vi "rule editor.vi"() -> (0 "output descriptions out":string[][](array[string]), 1 "State names":string[](array[string]), 3 "rule file":path, 4 "output descriptions out 2":string[][](array[string]))   [LabVIEW 2015]
uses:
  rule.ctl
  condition.ctl
  greater or less.ctl
  toolbar icons/Save configuration.ctl
  toolbar icons/open configuration.ctl
  toolbar icons/help.ctl
  variable setpoint.ctl
  data ave interval.ctl
  type specifier for control code.ctl
  rules.ctl
  State rules.ctl
  Output control.ctl
  logic buffer cmd.ctl
  Calibration and Function folders.ctl
  DAQ configuration/Sensor buffer command.ctl
  calibration/Shared Data/share data command.ctl
  <vilib>/Platform/browser.llb/Open URL in Default Browser (string).vi
panel:
  in  "new element/subarray":T1={"name"="new set point", "unit"="", "value"=0.0, "Type"=enum."Constant", "variable"={"selected sensors"=[], "selected set points"=[], "VI"=path "", "Data average interval"=0.0, "code ref"=refnum}} {"value" format="%#_6p"; "variable"."Data average interval" min=0.0 format="%^#_3g"}
  in  "Tab Control":enum32{"Set Points", "Rules & Outputs"}(tab)
  in  "Delete all set points":bool
  in  "Configure Function":bool
  in  "Calculate set point":bool
  out "Required Sensors":i32(listbox)
  out "Required Set Points":i32(listbox)
  out "code match":bool
  out "data match":bool
  in  "S P & V definitions":T1[](array[typedef]) {"value" format="%#_6p"; "variable"."Data average interval" min=0.0 format="%^#_3g"}
  in  "delete set point":bool
  in  "add set point after":bool
  in  "Set Points and Variables List":i32(listbox)=1
  in  "Tab states and rules":enum32{"Rules", "Outputs"}(tab)
  in  "Rules":T4=[{"state rules"=[{"next state"=0, "conditions"=[], "number of conditions"=0, "Rule name"=""}, {"next state"=1, "conditions"=[{"> or <"=FALSE, "set point"=500, "sensors and variables"=0, "Data average interval"=0.0}], "number of conditions"=1, "Rule name"=""}, {"next state"=1, "conditions"=[{"> or <"=FALSE, "set point"=10, "sensors and variables"=0, "Data average interval"=0.0}, {"> or <"=FALSE, "set point"=10, "sensors and variables"=0, "Data average interval"=0.0}, {"> or <"=TRUE, "set point"=20, "sensors and variables"=0, "Data average interval"=0.0}, {"> or <"=TRUE, "set point"=500, "sensors and variables"=0, "Data average interval"=0.0}], "number of conditions"=4, "Rule name"=""}], "State name"=""}, {"state rules"=[{"next state"=1, "conditions"=[{"> or <"=FALSE, "set point"=0, "sensors and variables"=0, "Data average interval"=0.0}], "number of conditions"=1, "Rule name"=""}, {"next state"=0, "conditions"=[{"> or <"=FALSE, "set point"=0, "sensors and variables"=0, "Data average interval"=0.0}], "number of conditions"=4, "Rule name"=""}], "State name"=""}] {"state rules"."number of conditions" min=1 step=1; "state rules"."conditions"."Data average interval" min=0.0 format="%^#_3g"; "state rules"."conditions"."sensors and variables" items=["Elapsed time in current state"]; "state rules"."conditions"."set point" items=["OFF", "ON"]; "state rules"."next state" items=["OFF"]}
  in  "output descriptions":string[][](array[string])
  in  "output settings":T9 items=["OFF", "ON"]
  in  "delete rule":bool
  in  "add rule after":bool
  in  "Rule List":i32(listbox)
  in  "delete state":bool
  in  "add state after":bool
  in  "State List":i32(listbox)
  in  "Help Button":T10
  out "Sensor names":string[](array[string])
  in  "Open logic":T11
  in  "Save logic":T12
  in  "new rule":cluster{"state rules":T6[], "State name":string}={"state rules"=[{"next state"=0, "conditions"=[{"> or <"=FALSE, "set point"=0, "sensors and variables"=0, "Data average interval"=0.0}], "number of conditions"=1, "Rule name"="New Rule"}], "State name"="New State"} {"state rules"."number of conditions" min=1 step=1; "state rules"."conditions"."Data average interval" min=0.0 format="%^#_3g"; "state rules"."conditions"."sensors and variables" items=["Elapsed time in current state"]; "state rules"."next state" items=["john", "dick"]}
  in  "OK Button":bool
  out "Unit":string[](array[string])
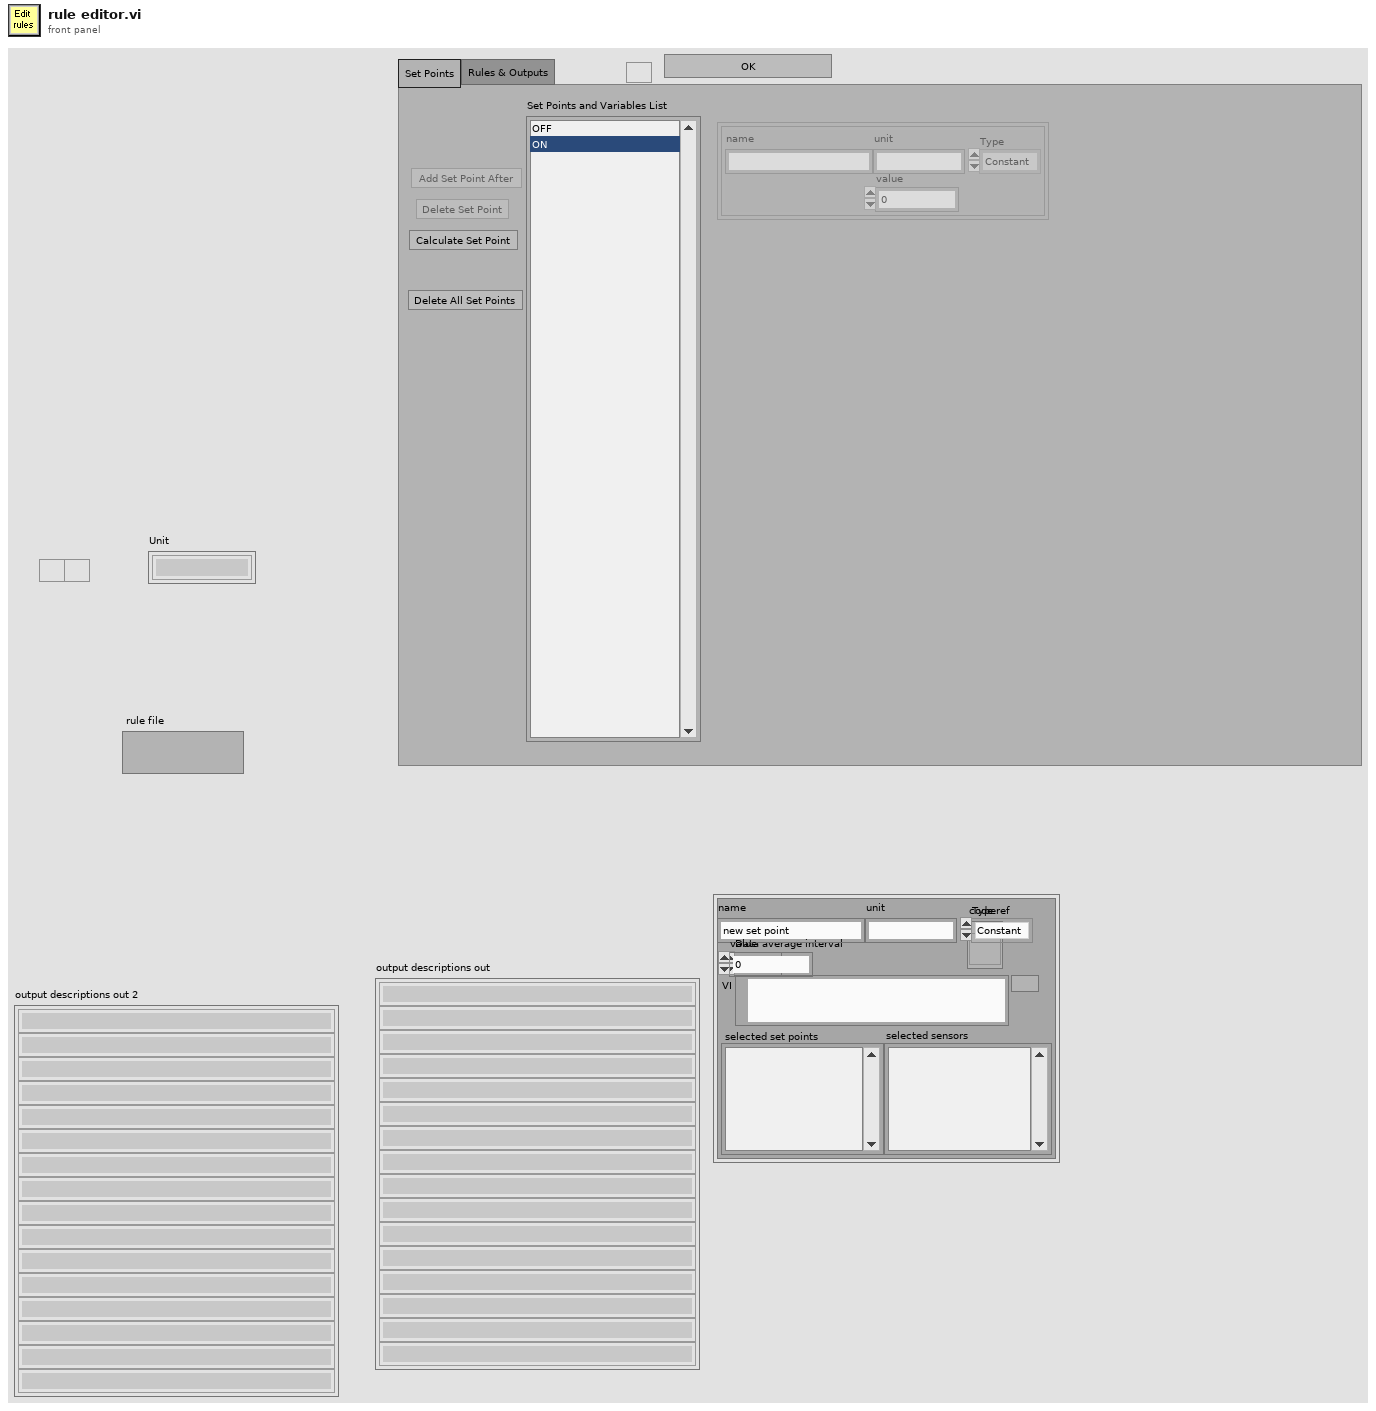
[diagram p1: front panel]
types:
  T1 = typedef "variable setpoint.ctl" = cluster{"name":string, "unit":string, "value":dbl, "Type":enum16{"Constant", "Variable"}, "variable":cluster{"selected sensors":i32[], "selected set points":i32[], "VI":path, "Data average interval":T2, "code ref":T3}}
  T2 = typedef "data ave interval.ctl" = dbl
  T3 = typedef "type specifier for control code.ctl" = refnum<vi>
  T4 = typedef "rules.ctl" = T5[]
  T5 = typedef "State rules.ctl" = cluster{"state rules":T6[], "State name":string}
  T6 = typedef "rule.ctl" = cluster{"next state":u16, "conditions":T7[], "number of conditions":u8, "Rule name":string}
  T7 = typedef "condition.ctl" = cluster{"> or <":T8, "set point":i32, "sensors and variables":i32, "Data average interval":dbl}
  T8 = typedef "greater or less.ctl" = bool
  T9 = typedef "Output control.ctl" = u16[][]
  T10 = typedef "help.ctl" = bool
  T11 = typedef "open configuration.ctl" = bool
  T12 = typedef "Save configuration.ctl" = bool
  T13 = typedef "share data command.ctl" = enum16{"Initialize from ini", "Update ini", "Write data", "Read data", "List my data", "List shared data", "Close"}
  T14 = typedef "Sensor buffer command.ctl" = enum16{"read average", "read recent", "read all", "write", "set buffer size", "Read channel config", "Write channel config", "clear"}
  T15 = typedef "Calibration and Function folders.ctl" = enum16{"Sensors", "Functions", "Config File", "PublicAppFolder", "New ini File", "Set Config File", "Delete ini File"}
  T16 = typedef "logic buffer cmd.ctl" = enum16{"read", "write ouput settings", "write rules", "write setpoints", "write output descriptions", "write all", "calculate setpoints", "save", "open", "Load all setpoint code", "Load one setpoint code", "Configure one setpoint code"}
  T17 = typedef "setpoint match.ctl" = cluster{"required data":cluster{"Set Point names":string[], "required number of setpoints":u8, "required number of sensors":u8, "Sensor names":string[]}, "input match":bool, "code match":bool, "variable?":bool}
  T18 = typedef "Channel config.ctl" = cluster{"Channel Indices":T19[], "AI Max voltage":dbl[], "Calibration matrix":T20}
  T19 = typedef "channel identifier.ctl" = u16
  T20 = typedef "calib array.ctl" = T21[]
  T21 = typedef "conversion.ctl" = cluster{"conversion matrix":sgl[][], "units":string, "name":string, "scale type":T22, "offset (volts)":dbl, "second channel":i8, "correspondence table":T23, "offset (physical units)":dbl, "pH scale":T24, "D.O.":T25, "Photometer data":T26}
  T22 = typedef "scale type.ctl" = enum16{"Volts", "Polynomial", "Correspondence Table", "pH", "Dissolved Oxygen", "Quadratic", "Photometer"}
  T23 = typedef "correspondence table.ctl" = cluster{"physical units":dbl, "volts":dbl}[]
  T24 = typedef "pH scale.ctl" = cluster{"Buffers":cluster{"Buffer":dbl, "Calibrated":bool, "V/T":dbl}[], "Temperature":dbl}
  T25 = typedef "DO scale.ctl" = cluster{"Temperature":dbl, "K":dbl, "barometric pressure":dbl}
  T26 = typedef "Photometer calibration data.ctl" = cluster{"Dark Voltage":dbl, "Blank Voltage":dbl, "Standards":cluster{"Concentration":dbl, "Voltage":dbl}[]}
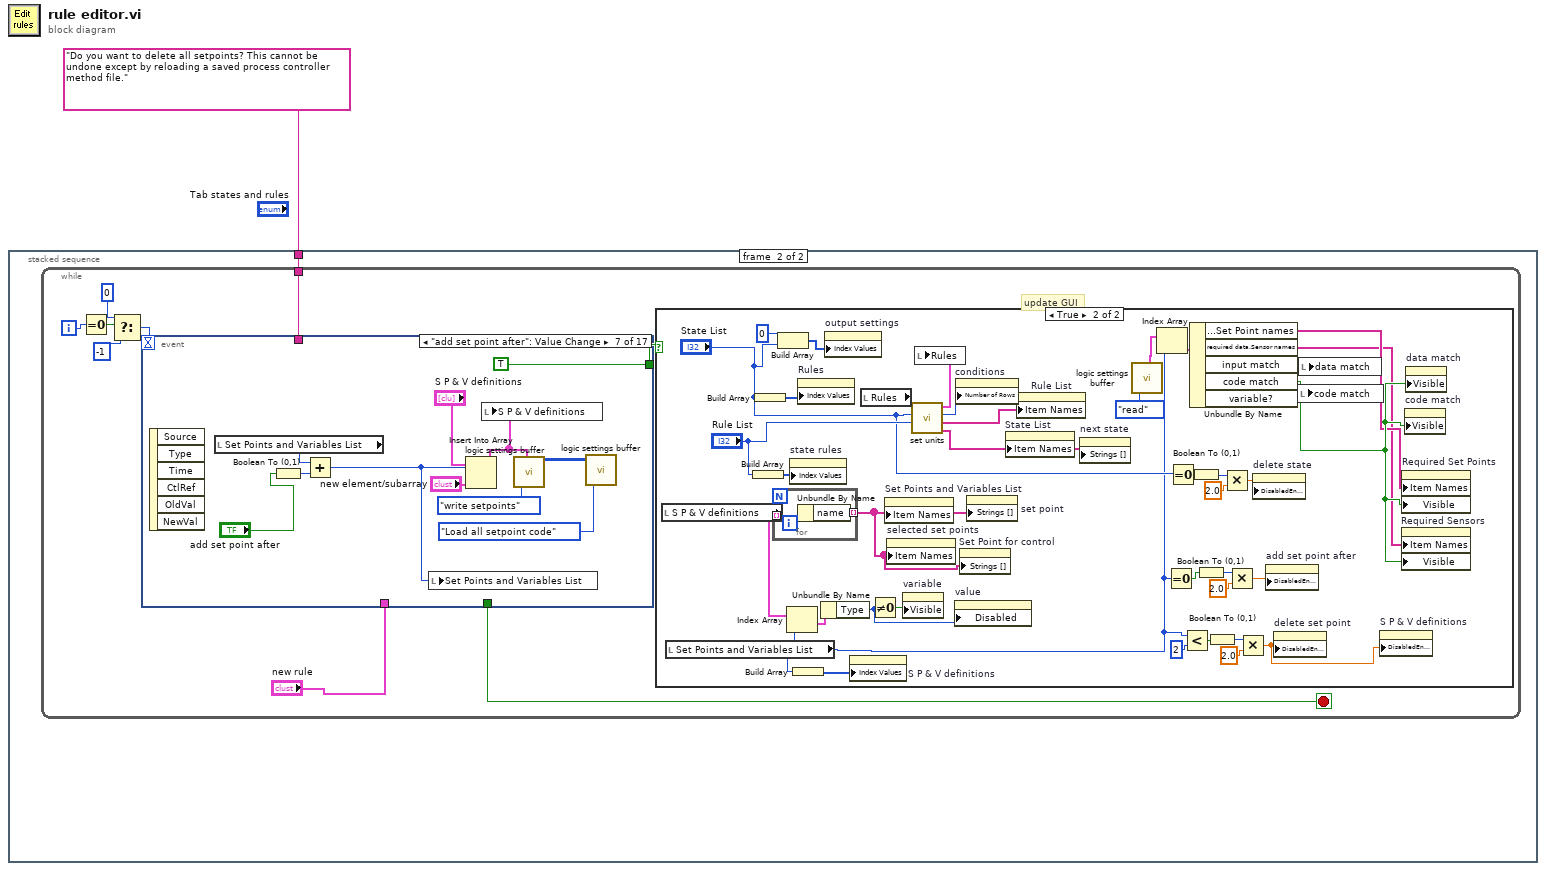
[diagram p0: block diagram]
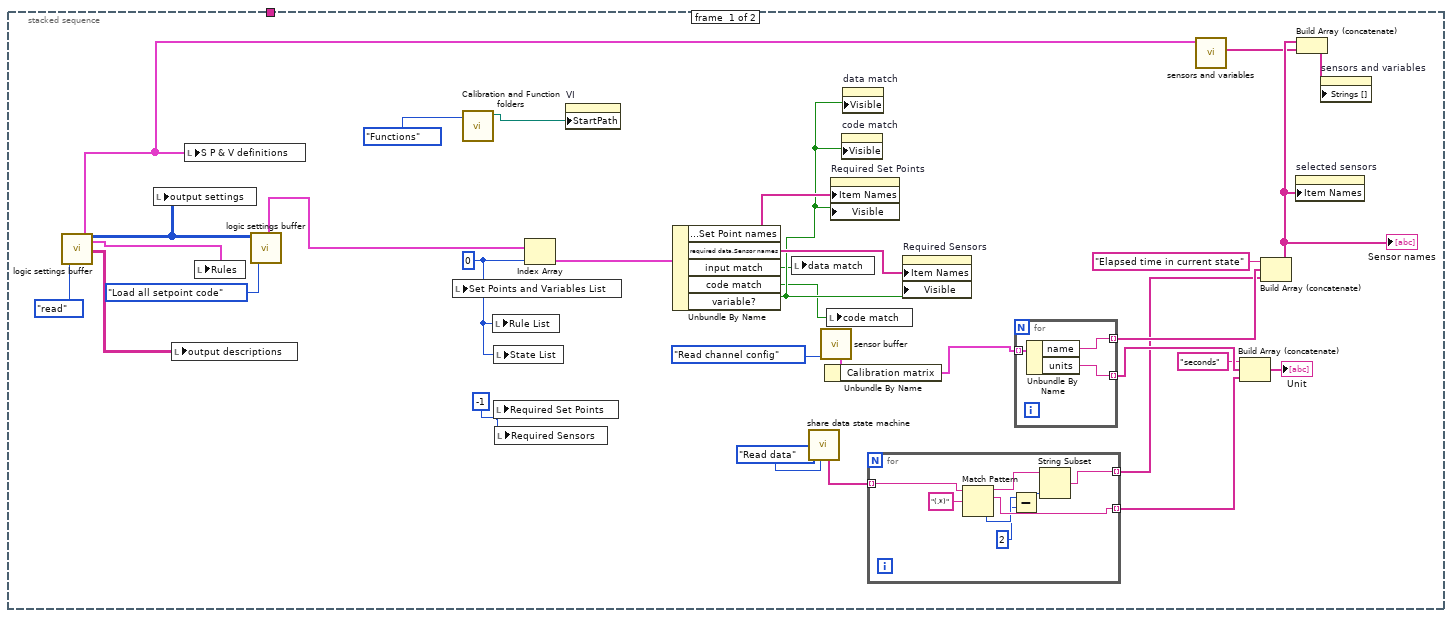
[diagram p2: hidden frame]
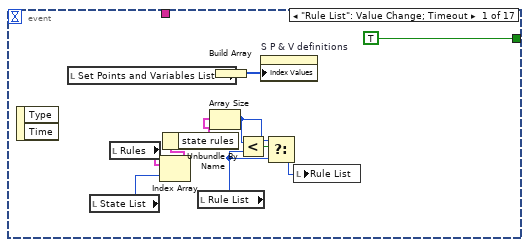
[diagram p4: hidden frame]
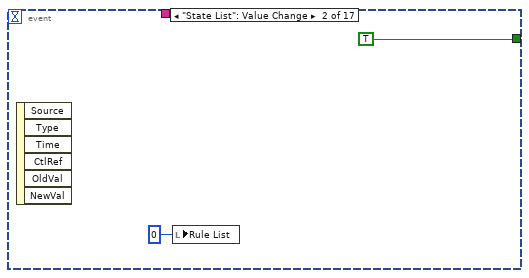
[diagram p5: hidden frame]
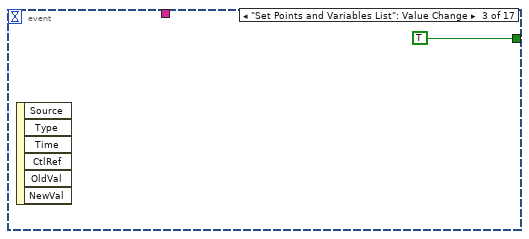
[diagram p6: hidden frame]
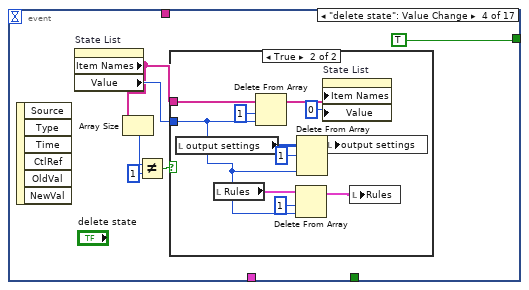
[diagram p7: hidden frame]
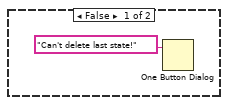
[diagram p8: hidden frame]
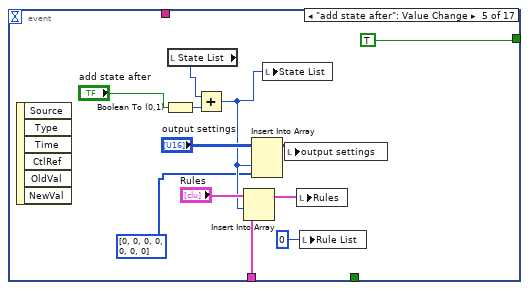
[diagram p9: hidden frame]
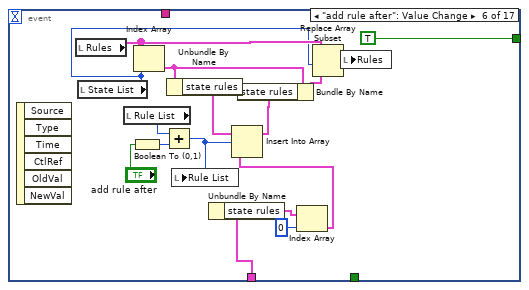
[diagram p10: hidden frame]
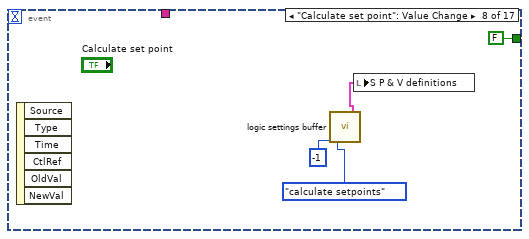
[diagram p11: hidden frame]
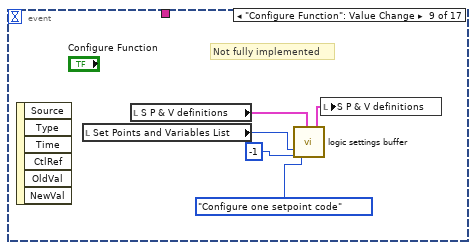
[diagram p12: hidden frame]
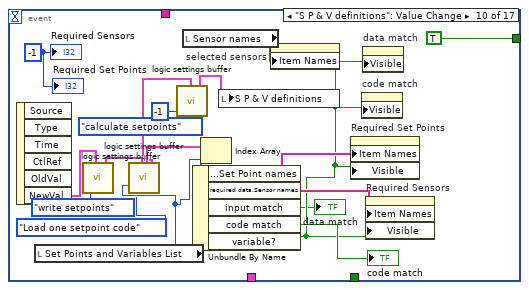
[diagram p13: hidden frame]
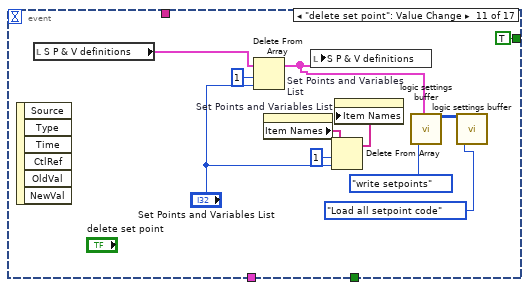
[diagram p14: hidden frame]
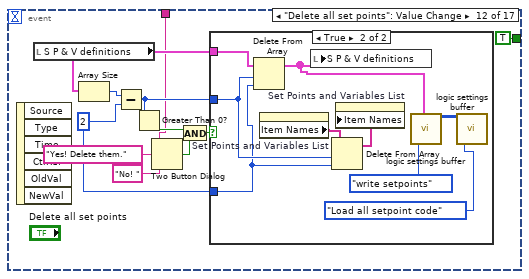
[diagram p15: hidden frame]
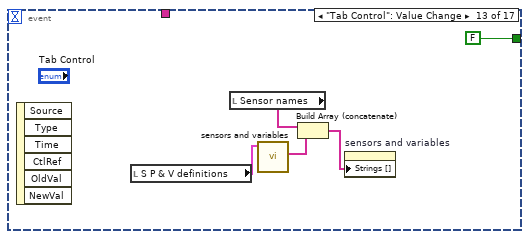
[diagram p17: hidden frame]
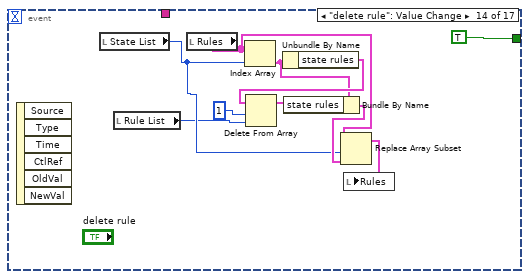
[diagram p18: hidden frame]
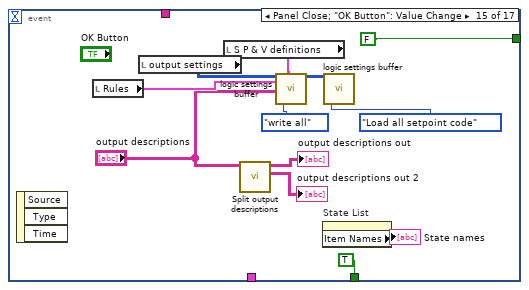
[diagram p19: hidden frame]
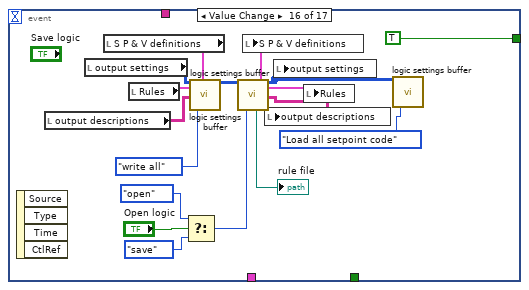
[diagram p20: hidden frame]
diagram:
  n1 = stacked-sequence {
    tunnel: "Do you want to delete all setpoints? This cannot be undone except by reloading a saved process controller method file." ("message") -> [_ w45]
    frame #0 {
      w20 = -1 ("Required Sensors")
      w19 = 0 ("Current Set Point")
      n2 = call "logic settings buffer.vi"("command"=logic_buffer_cmd."read") -> ("Set Points out"=w14:T1[], "ouput settings out"=w27:T9, "Rules out"=w30:T4, "output descriptions out"=w29:string[][])  [unwired: 11 in, 4 out]
      n3 = local write "output settings"(w27) -> ()
      n4 = local write "output descriptions"(w29) -> ()
      n5 = local write "S P & V definitions"(w14) -> ()
      n6 = local write "Rules"(w30) -> ()
      n7 = call "logic settings buffer.vi"("output settings"=w27, "command"=logic_buffer_cmd."Load all setpoint code") -> ("Setpoint match"=w15:T17[])  [unwired: 10 in, 7 out]
      n8 = local write "Set Points and Variables List"(w19) -> ()
      n9 = call "Calibration and Function folders.vi"("Folder"=Calibration_and_Function_folders."Functions") -> ("Selected Folder"=w8:path)  [unwired: 9 in, 1 out]
      n10 = local write "Rule List"(w19) -> ()
      n11 = local write "State List"(w19) -> ()
      n12 = local write "Required Set Points"(w20) -> ()
      n13 = local write "Required Sensors"(w20) -> ()
      n14 = Index Array(array=w15, index=w19) -> (element=w24:T17)
      n15 = property on="VI" class="Path"("StartPath"=w8) -> ()  [unwired: 2 in, 2 out]
      n16 = Unbundle By Name(w24) -> ("required data.Set Point names"=w26:string[], "required data.Sensor names"=w25:string[], "input match"=w21:bool, "code match"=w22:bool, "variable?"=w23:bool)
      n17 = local write "data match"(w21) -> ()
      n18 = call "share data state machine.vi"("Share data command"=share_data_command."Read data") -> ("Shared data names (unit)"=w2:string[])  [unwired: 4 in, 6 out]
      n19 = call "sensor buffer.vi"("command"=Sensor_buffer_command."Read channel config") -> ("Channel Config out"=w3:T18)  [unwired: 6 in, 4 out]
      n20 = Unbundle By Name(w3) -> ("Calibration matrix"=w9:T20)
      n21 = local write "code match"(w22) -> ()
      n22 = property on="Required Set Points" class="LstBox (strict)"("Item Names"=w26, "Visible"=w23) -> ()  [unwired: 2 in, 2 out]
      n23 = property on="code match" class="Bool (strict)"("Visible"=w23) -> ()  [unwired: 2 in, 2 out]
      n24 = property on="data match" class="Bool (strict)"("Visible"=w23) -> ()  [unwired: 2 in, 2 out]
      n25 = for {
        tunnel: w2 -> [w40] mode=indexing
        tunnel: [w39] -> w5 mode=indexing
        tunnel: [w38] -> w4 mode=indexing
        n26 = Match Pattern(string=w40, regular expression="(.*)") -> (before substring=w37:string, match substring=w39:string, offset past match=w36:i32)  [unwired: 1 in, 1 out]
        n27 = Subtract(x=w36, y=2) -> (x-y=w34:i32)
        n28 = String Subset(string=w37, length (rest)=w34) -> (substring=w38:string)  [unwired: 1 in]
      }
      n29 = property on="Required Sensors" class="LstBox (strict)"("Item Names"=w25, "Visible"=w23) -> ()  [unwired: 2 in, 2 out]
      n30 = for {
        tunnel: w9 -> [w44] mode=indexing
        tunnel: [w43] -> w33 mode=indexing
        tunnel: [w42] -> w18 mode=indexing
        n31 = Unbundle By Name(w44) -> ("name"=w42:string, "units"=w43:string)
      }
      n32 = call "sensors and variables.vi"("S P & V definitions"=w14) -> ("Variable names"=w11:string[])  [unwired: 6 in, 4 out]
      n33 = Build Array (concatenate)("seconds" ("name"), w33, w5) -> (→"Unit":string[])
      n34 = Build Array (concatenate)("Elapsed time in current state" ("name"), w18, w4) -> (w12:string[])
      "Sensor names" <- w12
      n35 = property on="selected sensors" class="LstBox (strict)"("Item Names"=w12) -> ()  [unwired: 2 in, 2 out]
      n36 = Build Array (concatenate)(w12, w11) -> (w13:string[])
      n37 = property on="sensors and variables" class="Ring (strict)"("Strings []"=w13) -> ()  [unwired: 2 in, 2 out]
    }
    frame #1 {
      n38 = while {
        tunnel: w45 -> [w46]
        i -> [w53]
        stop <- w54 stop-if-true
        # "update GUI"
        n39 = Equal To 0?(x=w53) -> (x = 0?=w52:bool)
        n40 = Select(t=0, s=w52, f=-1) -> (s? t:f=w47:i32)
        n41 = event shown="[6] \"add set point after\": Value Change" {
          selector: _ -> [_ _ _ _ _ _ _ _ _ _ _ _ _ _ _ _ _]
          dyn-events: _ -> [_ _ _ _ _ _ _ _ _ _ _ _ _ _ _ _ _]
          timeout: w47 -> [_ _ _ _ _ _ _ _ _ _ _ _ _ _ _ _ _]
          tunnel: [_ _ _ _ _ _ _ _ _ _ _ _ _ _ TRUE _ _] -> w54
          tunnel: [TRUE TRUE TRUE TRUE TRUE TRUE TRUE FALSE _ TRUE TRUE TRUE FALSE TRUE FALSE TRUE _] -> w49
          tunnel: "new rule" -> [_ _ _ _ w133 w146 _ _ _ _ _ _ _ _ _ _ _]
          tunnel: w46 -> [_ _ _ _ _ _ _ _ _ _ _ w208 _ _ _ _ _]
          event "Rule List": Value Change; Timeout {
            n42 = event-data() -> ()  [unwired: 1 in, 2 out]
            n43 = local read "Set Points and Variables List"() -> (w97:i32)
            n44 = local read "State List"() -> (w101:i32)
            n45 = local read "Rules"() -> (w98:T4)
            n46 = Index Array(array=w98, index=w101) -> (element=w100:T5)
            n47 = Unbundle By Name(w100) -> ("state rules"=w99:T6[])
            n48 = local read "Rule List"() -> (w102:i32)
            n49 = Array Size(array=w99) -> (size(s)=w103:i32)
            n50 = Build Array(w97) -> (w96:i32[])
            n51 = Less?(x=w103, y=w102) -> (x < y?=w105:bool)
            n52 = property on="S P & V definitions" class="Arr (strict)"("Index Values"=w96) -> ()  [unwired: 2 in, 2 out]
            n53 = Select(t=w103, s=w105, f=w102) -> (s? t:f=w104:i32)
            n54 = local write "Rule List"(w104) -> ()
          }
          event "State List": Value Change {
            n55 = event-data() -> ()  [unwired: 1 in, 6 out]
            n56 = local write "Rule List"(0 ("Current Rule")) -> ()
          }
          event "Set Points and Variables List": Value Change {
            n57 = event-data() -> ()  [unwired: 1 in, 6 out]
          }
          event "delete state": Value Change {
            n58 = event-data() -> ()  [unwired: 1 in, 6 out]
            n59 = property on="State List" class="LstBox (strict)"() -> ("Item Names"=w113:string[], "Value"=w114:i32)  [unwired: 2 in, 2 out]
            n60 = Array Size(array=w113) -> (size(s)=w111:i32)
            n61 = Not Equal?(x=w111, y=1) -> (x != y?=w112:bool)
            n62 = case shown="True" w112 {
              tunnel: w113 -> [_ w123]
              tunnel: w114 -> [_ w117]
              frame False {
                n63 = One Button Dialog(message="Can't delete last state!") -> ()  [unwired: 1 in, 1 out]
              }
              frame True {
                n64 = local read "output settings"() -> (w126:T9)
                n65 = local read "Rules"() -> (w121:T4)
                n66 = Delete From Array(array=w123, length=1, index=w117) -> (array with subset deleted=w119:string[])  [unwired: 1 out]
                n67 = Delete From Array(array=w121, length=1, index=w117) -> (array with subset deleted=w120:T4)  [unwired: 1 out]
                n68 = Delete From Array(array=w126, length=1, index (col)=w117) -> (array with subset deleted=w127:T9)  [unwired: 1 in, 1 out]
                n69 = property on="State List" class="LstBox (strict)"("Item Names"=w119, "Value"=0 ("Current State")) -> ()  [unwired: 2 in, 2 out]
                n70 = local write "output settings"(w127) -> ()
                n71 = local write "Rules"(w120) -> ()
              }
            }
          }
          event "add state after": Value Change {
            n72 = event-data() -> ()  [unwired: 1 in, 6 out]
            n73 = Boolean To (0,1)(Boolean="add state after") -> (0, 1=w138:i16)
            n74 = local read "State List"() -> (w132:i32)
            n75 = Add(x=w132, y=w138) -> (x+y=w129:i32)
            n76 = Insert Into Array(array="Rules", index=w129, new element=w133) -> (w136:T4)
            n77 = Insert Into Array(array="output settings", index (col)=w129, new element=u16[] [0, 0, 0, 0, 0, 0, 0] ("new element/subarray")) -> (w139:T9)  [unwired: 1 in]
            n78 = local write "State List"(w129) -> ()
            n79 = local write "output settings"(w139) -> ()
            n80 = local write "Rules"(w136) -> ()
            n81 = local write "Rule List"(0 ("Current Rule")) -> ()
          }
          event "add rule after": Value Change {
            n82 = event-data() -> ()  [unwired: 1 in, 6 out]
            n83 = local read "Rules"() -> (w142:T4)
            n84 = local read "State List"() -> (w141:i32)
            n85 = local read "Rule List"() -> (w152:i32)
            n86 = Boolean To (0,1)(Boolean="add rule after") -> (0, 1=w153:i16)
            n87 = Index Array(array=w142, index=w141) -> (element=w150:T5)
            n88 = Add(x=w152, y=w153) -> (x+y=w140:i32)
            n89 = Unbundle By Name(w150) -> ("state rules"=w149:T6[])
            n90 = local write "Rule List"(w140) -> ()
            n91 = Unbundle By Name(w146) -> ("state rules"=w145:T6[])
            n92 = Index Array(array=w145, index=0) -> (element=w144:T6)
            n93 = Insert Into Array(array=w149, index=w140, new element=w144) -> (w148:T6[])
            n94 = Bundle By Name(cluster=w150, "state rules"=w148) -> (w147:T5)
            n95 = Replace Array Subset(array=w142, new element=w147, index=w141) -> (w151:T4)
            n96 = local write "Rules"(w151) -> ()
          }
          event "add set point after": Value Change {
            n97 = event-data() -> ()  [unwired: 1 in, 6 out]
            n98 = local read "Set Points and Variables List"() -> (w165:i32)
            n99 = Boolean To (0,1)(Boolean="add set point after") -> (0, 1=w166:i16)
            n100 = Add(x=w165, y=w166) -> (x+y=w163:i32)
            n101 = local write "Set Points and Variables List"(w163) -> ()
            n102 = Insert Into Array(array="S P & V definitions", index=w163, new element="new element/subarray") -> (w160:T1[])
            n103 = local write "S P & V definitions"(w160) -> ()
            n104 = call "logic settings buffer.vi"("command"=logic_buffer_cmd."write setpoints", "Set Points"=w160) -> ("ouput settings out"=w158:T9)  [unwired: 10 in, 7 out]
            n105 = call "logic settings buffer.vi"("output settings"=w158, "command"=logic_buffer_cmd."Load all setpoint code") -> ()  [unwired: 10 in, 8 out]
          }
          event "Calculate set point": Value Change {
            n106 = event-data() -> ()  [unwired: 1 in, 6 out]
            n107 = call "logic settings buffer.vi"("Plant  state"=-1, "command"=logic_buffer_cmd."calculate setpoints") -> ("Set Points out"=w168:T1[])  [unwired: 10 in, 7 out]
            n108 = local write "S P & V definitions"(w168) -> ()
          }
          event "Configure Function": Value Change {
            # "Not fully implemented"
            n109 = event-data() -> ()  [unwired: 1 in, 6 out]
            n110 = local read "Set Points and Variables List"() -> (w171:i32)
            n111 = local read "S P & V definitions"() -> (w173:T1[])
            n112 = call "logic settings buffer.vi"("index"=w171, "Plant  state"=-1, "command"=logic_buffer_cmd."Configure one setpoint code", "Set Points"=w173) -> ("Set Points out"=w175:T1[])  [unwired: 8 in, 7 out]
            n113 = local write "S P & V definitions"(w175) -> ()
          }
          event "S P & V definitions": Value Change {
            w190 = -1 ("Required Sensors")
            n114 = event-data() -> ("NewVal"=w181:T1[])  [unwired: 1 in, 5 out]
            n115 = local read "Set Points and Variables List"() -> (w187:i32)
            n116 = call "logic settings buffer.vi"("command"=logic_buffer_cmd."write setpoints", "Set Points"=w181) -> ("Set Points out"=w188:T1[])  [unwired: 10 in, 7 out]
            n117 = call "logic settings buffer.vi"("index"=w187, "command"=logic_buffer_cmd."Load one setpoint code", "Set Points"=w188) -> ("Setpoint match"=w186:T17[], "Set Points out"=w179:T1[])  [unwired: 9 in, 6 out]
            n118 = call "logic settings buffer.vi"("Plant  state"=-1, "command"=logic_buffer_cmd."calculate setpoints", "Set Points"=w179) -> ("Set Points out"=w178:T1[])  [unwired: 9 in, 7 out]
            n119 = local read "Sensor names"() -> (w193:string[])
            n120 = Index Array(array=w186, index=w187) -> (element=w185:T17)
            n121 = Unbundle By Name(w185) -> ("required data.Set Point names"=w192:string[], "required data.Sensor names"=w191:string[], "input match"=→"data match":bool, "code match"=→"code match":bool, "variable?"=w183:bool)
            n122 = local write "S P & V definitions"(w178) -> ()
            n123 = property on="selected sensors" class="LstBox (strict)"("Item Names"=w193) -> ()  [unwired: 2 in, 2 out]
            n124 = property on="Required Set Points" class="LstBox (strict)"("Item Names"=w192, "Visible"=w183) -> ()  [unwired: 2 in, 2 out]
            n125 = property on="code match" class="Bool (strict)"("Visible"=w183) -> ()  [unwired: 2 in, 2 out]
            n126 = property on="data match" class="Bool (strict)"("Visible"=w183) -> ()  [unwired: 2 in, 2 out]
            n127 = property on="Required Sensors" class="LstBox (strict)"("Item Names"=w191, "Visible"=w183) -> ()  [unwired: 2 in, 2 out]
            "Required Set Points" <- w190
            "Required Sensors" <- w190
          }
          event "delete set point": Value Change {
            n128 = event-data() -> ()  [unwired: 1 in, 6 out]
            n129 = local read "S P & V definitions"() -> (w205:T1[])
            n130 = Delete From Array(array=w205, length=1, index="Set Points and Variables List") -> (array with subset deleted=w198:T1[])  [unwired: 1 out]
            n131 = property on="Set Points and Variables List" class="LstBox (strict)"() -> ("Item Names"=w202:string[])  [unwired: 2 in, 2 out]
            n132 = local write "S P & V definitions"(w198) -> ()
            n133 = Delete From Array(array=w202, length=1, index="Set Points and Variables List") -> (array with subset deleted=w201:string[])  [unwired: 1 out]
            n134 = property on="Set Points and Variables List" class="LstBox (strict)"("Item Names"=w201) -> ()  [unwired: 2 in, 2 out]
            n135 = call "logic settings buffer.vi"("command"=logic_buffer_cmd."write setpoints", "Set Points"=w198) -> ("ouput settings out"=w195:T9)  [unwired: 10 in, 7 out]
            n136 = call "logic settings buffer.vi"("output settings"=w195, "command"=logic_buffer_cmd."Load all setpoint code") -> ()  [unwired: 10 in, 8 out]
          }
          event "Delete all set points": Value Change {
            w213 = 2 ("y")
            n137 = event-data() -> ()  [unwired: 1 in, 6 out]
            n138 = local read "S P & V definitions"() -> (w215:T1[])
            n139 = Array Size(array=w215) -> (size(s)=w214:i32)
            n140 = Subtract(x=w214, y=w213) -> (x-y=w211:i32)
            n141 = Greater Than 0?(x=w211) -> (x > 0?=w210:bool)
            n142 = Two Button Dialog(message=w208, 1:"No! " ("F button name (\"Cancel\")"), 2:"Yes! Delete them." ("T button name (\"OK\")")) -> (T button?=w212:bool)
            n143 = And(x=w210, y=w212) -> (x .and. y?=w209:bool)
            n144 = case shown="True" w209 {
              tunnel: w215 -> [_ w219]
              tunnel: w211 -> [_ w218]
              tunnel: w213 -> [_ w217]
              frame False {
              }
              frame True {
                n145 = Delete From Array(array=w219, length=w218, index=w217) -> (array with subset deleted=w225:T1[])  [unwired: 1 out]
                n146 = property on="Set Points and Variables List" class="LstBox (strict)"() -> ("Item Names"=w221:string[])  [unwired: 2 in, 2 out]
                n147 = local write "S P & V definitions"(w225) -> ()
                n148 = Delete From Array(array=w221, length=w218, index=w217) -> (array with subset deleted=w220:string[])  [unwired: 1 out]
                n149 = property on="Set Points and Variables List" class="LstBox (strict)"("Item Names"=w220) -> ()  [unwired: 2 in, 2 out]
                n150 = call "logic settings buffer.vi"("command"=logic_buffer_cmd."write setpoints", "Set Points"=w225) -> ("ouput settings out"=w222:T9)  [unwired: 10 in, 7 out]
                n151 = call "logic settings buffer.vi"("output settings"=w222, "command"=logic_buffer_cmd."Load all setpoint code") -> ()  [unwired: 10 in, 8 out]
              }
            }
          }
          event "Tab Control": Value Change {
            n152 = event-data() -> ()  [unwired: 1 in, 6 out]
            n153 = local read "S P & V definitions"() -> (w229:T1[])
            n154 = local read "Sensor names"() -> (w227:string[])
            n155 = call "sensors and variables.vi"("S P & V definitions"=w229) -> ("Variable names"=w228:string[])  [unwired: 6 in, 4 out]
            n156 = Build Array (concatenate)(w227, w228) -> (w226:string[])
            n157 = property on="sensors and variables" class="Ring (strict)"("Strings []"=w226) -> ()  [unwired: 2 in, 2 out]
          }
          event "delete rule": Value Change {
            n158 = event-data() -> ()  [unwired: 1 in, 6 out]
            n159 = local read "State List"() -> (w232:i32)
            n160 = local read "Rule List"() -> (w231:i32)
            n161 = local read "Rules"() -> (w236:T4)
            n162 = Index Array(array=w236, index=w232) -> (element=w238:T5)
            n163 = Unbundle By Name(w238) -> ("state rules"=w239:T6[])
            n164 = Delete From Array(array=w239, length=1, index=w231) -> (array with subset deleted=w237:T6[])  [unwired: 1 out]
            n165 = Bundle By Name(cluster=w238, "state rules"=w237) -> (w234:T5)
            n166 = Replace Array Subset(array=w236, new element=w234, index=w232) -> (w235:T4)
            n167 = local write "Rules"(w235) -> ()
          }
          event Panel Close; "OK Button": Value Change {
            n168 = event-data() -> ()  [unwired: 1 in, 3 out]
            n169 = local read "Rules"() -> (w248:T4)
            n170 = local read "output settings"() -> (w249:T9)
            n171 = local read "S P & V definitions"() -> (w247:T1[])
            n172 = call "Split output descriptions.vi"("output descriptions combined"="output descriptions") -> ("output descriptions 2"=→"output descriptions out 2":string[][], "output descriptions"=→"output descriptions out":string[][])  [unwired: 9 in]
            n173 = call "logic settings buffer.vi"("output settings"=w249, "Rules"=w248, "output descriptions"="output descriptions", "command"=logic_buffer_cmd."write all", "Set Points"=w247) -> ("ouput settings out"=w244:T9)  [unwired: 7 in, 7 out]
            n174 = property on="State List" class="LstBox (strict)"() -> ("Item Names"=→"State names":string[])  [unwired: 2 in, 2 out]
            n175 = call "logic settings buffer.vi"("output settings"=w244, "command"=logic_buffer_cmd."Load all setpoint code") -> ()  [unwired: 10 in, 8 out]
          }
          event Value Change {
            n176 = event-data() -> ()  [unwired: 1 in, 4 out]
            n177 = local read "output descriptions"() -> (w256:string[][])
            n178 = local read "output settings"() -> (w259:T9)
            n179 = local read "S P & V definitions"() -> (w260:T1[])
            n180 = local read "Rules"() -> (w258:T4)
            n181 = Select(t=logic_buffer_cmd."open" ("command"), s="Open logic", f=logic_buffer_cmd."save" ("command")) -> (s? t:f=w266:T16)
            n182 = call "logic settings buffer.vi"("output settings"=w259, "Rules"=w258, "output descriptions"=w256, "command"=logic_buffer_cmd."write all", "Set Points"=w260) -> ("ouput settings out"=w262:T9)  [unwired: 7 in, 7 out]
            n183 = call "logic settings buffer.vi"("output settings"=w262, "command"=w266) -> ("Set Points out"=w265:T1[], "rule file out"=→"rule file":path, "ouput settings out"=w254:T9, "Rules out"=w264:T4, "output descriptions out"=w253:string[][])  [unwired: 10 in, 3 out]
            n184 = local write "S P & V definitions"(w265) -> ()
            n185 = local write "output descriptions"(w253) -> ()
            n186 = local write "output settings"(w254) -> ()
            n187 = local write "Rules"(w264) -> ()
            n188 = call "logic settings buffer.vi"("output settings"=w254, "command"=logic_buffer_cmd."Load all setpoint code") -> ()  [unwired: 10 in, 8 out]
          }
          event Value Change {
            n189 = event-data() -> ()  [unwired: 1 in, 4 out]
            n190 = call-poly <vilib>:"Open URL in Default Browser.vi"("URL"="https://monroews.github.io/EnvEngLabTextbook/ProCoDA/ProCoDA.html#logic-states-and-outputs-config-edit-rules") -> ()  [unwired: 5 in, 2 out]
          }
        }
        n191 = case shown="True" w49 {
          frame False {
          }
          frame True {
            n192 = local read "S P & V definitions"() -> (w86:T1[])
            n193 = local read "Set Points and Variables List"() -> (w57:i32)
            n194 = Build Array("Rule List") -> (w93:i32[])
            n195 = Build Array("State List") -> (w84:i32[])
            n196 = for {
              tunnel: w86 -> [w95] mode=indexing
              tunnel: [w94] -> w81 mode=indexing
              n197 = Unbundle By Name(w95) -> ("name"=w94:string)
            }
            n198 = Build Array(0 ("element"), "State List") -> (w83:i32[])
            n199 = Index Array(array=w86, index=w57) -> (element=w85:T1)
            n200 = property on="state rules" class="Arr (strict)"("Index Values"=w93) -> ()  [unwired: 2 in, 2 out]
            n201 = Build Array(w57) -> (w87:i32[])
            n202 = property on="Rules" class="Arr (strict)"("Index Values"=w84) -> ()  [unwired: 2 in, 2 out]
            n203 = Unbundle By Name(w85) -> ("Type"=w79:enum16{"Constant", "Variable"})
            n204 = property on="output settings" class="Arr (strict)"("Index Values"=w83) -> ()  [unwired: 2 in, 2 out]
            n205 = property on="S P & V definitions" class="Arr (strict)"("Index Values"=w87) -> ()  [unwired: 2 in, 2 out]
            n206 = local read "Rules"() -> (w88:T4)
            n207 = Not Equal To 0?(x=w79) -> (x != 0?=w80:bool)
            n208 = property on="Set Points and Variables List" class="LstBox (strict)"("Item Names"=w81) -> ()  [unwired: 2 in, 2 out]
            n209 = property on="selected set points" class="LstBox (strict)"("Item Names"=w81) -> ()  [unwired: 2 in, 2 out]
            n210 = property on="variable" class="Clust (strict)"("Visible"=w80) -> ()  [unwired: 2 in, 2 out]
            n211 = call "set units.vi"("Current Rule"="Rule List", "Current State"="State List", "Rules"=w88) -> ("State names"=w89:string[], "Rule names"=w90:string[], "number of conditions"=w78:u8, "Rules out"=w92:T4)  [unwired: 1 in]
            n212 = local write "Rules"(w92) -> ()
            n213 = property on="value" class="DigNum (strict)"("Disabled"=w79) -> ()  [unwired: 2 in, 2 out]
            n214 = property on="conditions" class="Arr (strict)"("Number of Rows"=w78) -> ()  [unwired: 2 in, 2 out]
            n215 = property on="Set Point for control" class="Ring (strict)"("Strings []"=w81) -> ()  [unwired: 2 in, 2 out]
            n216 = property on="set point" class="Ring (strict)"("Strings []"=w81) -> ()  [unwired: 2 in, 2 out]
            n217 = property on="State List" class="LstBox (strict)"("Item Names"=w89) -> ()  [unwired: 2 in, 2 out]
            n218 = property on="Rule List" class="LstBox (strict)"("Item Names"=w90) -> ()  [unwired: 2 in, 2 out]
            n219 = property on="next state" class="Ring (strict)"("Strings []"=w89) -> ()  [unwired: 2 in, 2 out]
            n220 = call "logic settings buffer.vi"("command"=logic_buffer_cmd."read") -> ("Setpoint match"=w77:T17[])  [unwired: 11 in, 7 out]
            n221 = Index Array(array=w77, index=w57) -> (element=w75:T17)
            n222 = Equal To 0?(x=w57) -> (x = 0?=w58:bool)
            n223 = Equal To 0?(x="State List") -> (x = 0?=w66:bool)
            n224 = Less?(x=w57, y=2) -> (x < y?=w60:bool)
            n225 = Unbundle By Name(w75) -> ("required data.Set Point names"=w71:string[], "required data.Sensor names"=w70:string[], "input match"=w74:bool, "code match"=w73:bool, "variable?"=w72:bool)
            n226 = Boolean To (0,1)(Boolean=w66) -> (0, 1=w65:i16)
            n227 = Boolean To (0,1)(Boolean=w58) -> (0, 1=w62:i16)
            n228 = Boolean To (0,1)(Boolean=w60) -> (0, 1=w59:i16)
            n229 = Multiply(x=w65, y=2.0) -> (x*y=w64:dbl)
            n230 = Multiply(x=w62, y=2.0) -> (x*y=w56:dbl)
            n231 = Multiply(x=w59, y=2.0) -> (x*y=w55:dbl)
            n232 = property on="delete state" class="Bool"("DisabledEnum"=w64) -> ()  [unwired: 2 in, 2 out]
            n233 = property on="add set point after" class="Bool"("DisabledEnum"=w56) -> ()  [unwired: 2 in, 2 out]
            n234 = property on="delete set point" class="Bool"("DisabledEnum"=w55) -> ()  [unwired: 2 in, 2 out]
            n235 = local write "code match"(w73) -> ()
            n236 = local write "data match"(w74) -> ()
            n237 = property on="S P & V definitions" class="Arr (strict)"("DisabledEnum"=w55) -> ()  [unwired: 2 in, 2 out]
            n238 = property on="Required Set Points" class="LstBox (strict)"("Item Names"=w71, "Visible"=w72) -> ()  [unwired: 2 in, 2 out]
            n239 = property on="Required Sensors" class="LstBox (strict)"("Item Names"=w70, "Visible"=w72) -> ()  [unwired: 2 in, 2 out]
            n240 = property on="code match" class="Bool (strict)"("Visible"=w72) -> ()  [unwired: 2 in, 2 out]
            n241 = property on="data match" class="Bool (strict)"("Visible"=w72) -> ()  [unwired: 2 in, 2 out]
          }
        }
      }
    }
  }
